vi "Rerun_GCFS.vi"() -> ()   [LabVIEW 2024]
uses:
  RerunCluster_GCFS.ctl
  <vilib>/userDefined/High Color/IMAQdx.ctl
  <vilib>/vision/Image Controls.llb/IMAQ Image.ctl
  <vilib>/Platform/TimedLoop/XDataNode/timing_clust.ctl
  <vilib>/Platform/TimedLoop/XDataNode/nitl_modes.ctl
  <vilib>/Platform/TimedLoop/XDataNode/wakeup.ctl
  <vilib>/addons/_JKI Toolkits/State Machine/_JKI_lib_State_Machine.llb/Select State(s)_err__jki_lib_state_machine.vi
  <extravilib>/ChannelInstances/Tag-t'RerunCluster_GCFS.ctl'/Read With Abort.vi
  <extravilib>/ChannelInstances/Stream-c(t'IMAQ Image.ctl',str,a[.,.](str),a[.,.](str),bool)/Read With Abort.vi
  <extravilib>/ChannelInstances/Stream-c(t'IMAQ Image.ctl',str,a[.,.](str),a[.,.](str),bool)/Write With Abort.vi
  <extravilib>/ChannelInstances/Tag-t'RerunCluster_GCFS.ctl'/Write With Abort.vi
  <extravilib>/ChannelInstances/Stream-c(t'IMAQ Image.ctl',str,a[.,.](str),a[.,.](str),bool)/EndpointRead.vi
  <extravilib>/ChannelInstances/Stream-c(t'IMAQ Image.ctl',str,a[.,.](str),a[.,.](str),bool)/Endpoint.vi
  <extravilib>/ChannelInstances/Stream-c(t'IMAQ Image.ctl',str,a[.,.](str),a[.,.](str),bool)/Instantiate.vi
  <extravilib>/ChannelInstances/Tag-t'RerunCluster_GCFS.ctl'/Instantiate.vi
  <extravilib>/ChannelInstances/Tag-t'RerunCluster_GCFS.ctl'/EndpointRead.vi
  <extravilib>/ChannelInstances/Stream-c(t'IMAQ Image.ctl',str,a[.,.](str),a[.,.](str),bool)/)Channel.vi
  <resource>/ChannelSupport/_ChannelSupport/WaitIfNeeded.vi
  <vilib>/addons/_JKI Toolkits/State Machine/_JKI_lib_State_Machine.llb/Periodic Trigger__ogtk__JKI-SM__jki_lib_state_machine.vi
  <vilib>/Utility/file.llb/Read Delimited Spreadsheet (DBL).vi
  <vilib>/Utility/file.llb/Read Delimited Spreadsheet (string).vi
  <extravilib>/ChannelInstances/Tag-t'RerunCluster_GCFS.ctl'/Endpoint.vi
  <vilib>/platform/TimedLoop/XDataNode/XDataNode.xnode
  <vilib>/regexp/Match Regular Expression.xnode
  <vilib>/Platform/TimedLoop/XDataNode/XDNodeRunTimeDep.lvlib
  <extravilib>/ChannelInstances/Stream-c(t'IMAQ Image.ctl',str,a[.,.](str),a[.,.](str),bool).lvlib
  <extravilib>/ChannelInstances/Tag-t'RerunCluster_GCFS.ctl'.lvlib
panel:
  out "Number of droplets":i32
  out "Droplet messurments":dbl[][](array[numeric])
  in  "Done":bool
  out "Timestamps and temp data":string[][](array[string])
  out "Sample Name":string
  out "Image":T1(plugin-control)
  in  "Active":bool
  in  "Load Rerun":bool
  out "Save loop":i32
  out "Frezz Image":T1(plugin-control)
  in  "Freezing value":sgl=250.0
  out "Temperature":dbl
  out "Data Loop":i32
  out "Statusstring":string
  in  "Exit":bool
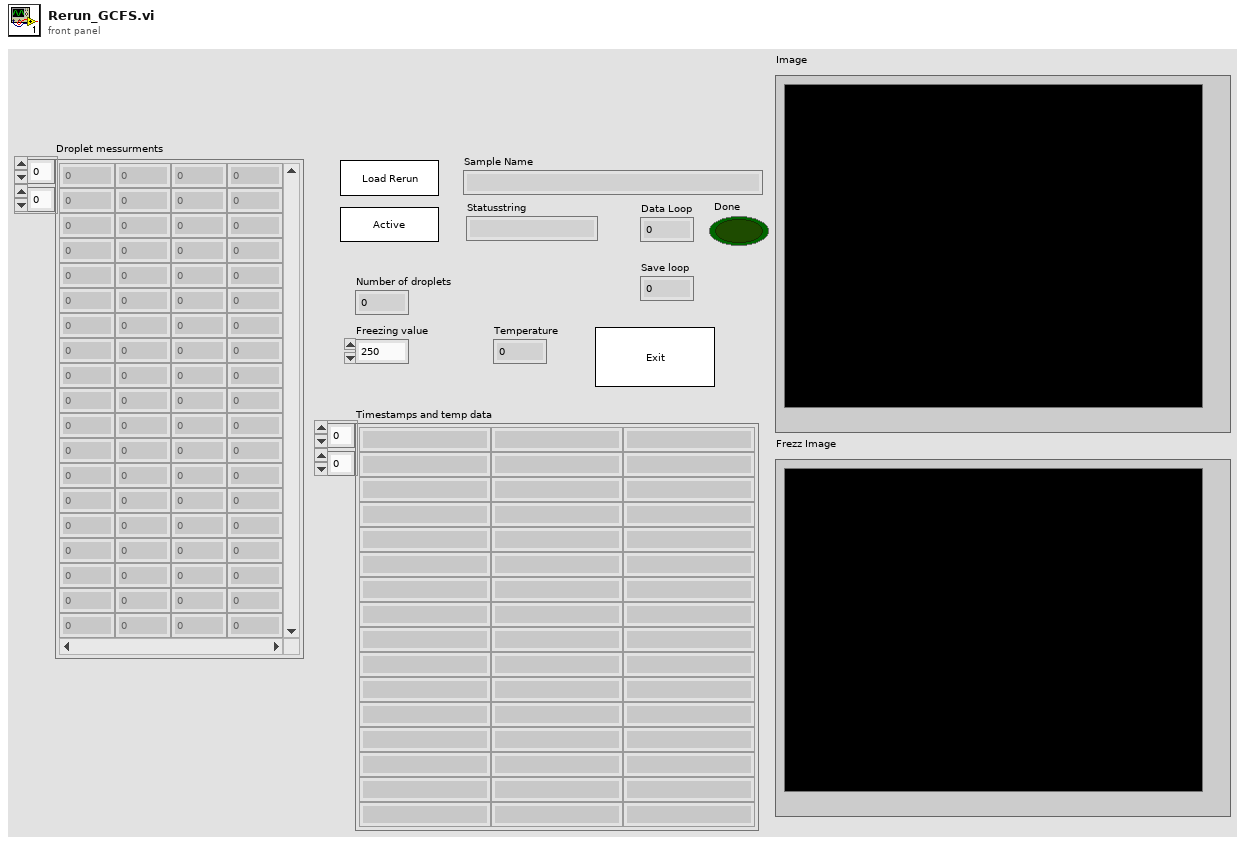
[diagram p1: front panel]
types:
  T1 = typedef "IMAQ Image.ctl" = refnum<image>
  T2 = typedef "RerunCluster_GCFS.ctl" = cluster{"Core":cluster{"Current VI Reference":refnum<vi>, "Close Panel on Exit?":bool}, "Your Boolean data":bool, "Your string data":string, "Camera Cluster":cluster{"Session":T3, "Image":T1, "Position Image":T1, "PixelVal Image":T1, "Position Image Rings":T1, "Lable Image":T1, "Merged Image":T1}, "Data In Cluster":cluster{"Images":cluster{"Position Image path":path, "Sample folder path":path, "Rerun Folder path":path, "Rerun pos.img. path":path}, "Sample Name":string, "Rerun Time":string, "Freezing value":sgl, "Number of images":i32}, "Active":bool, "Ready":bool, "Exit":bool, "Program_Start":string, "Data Out Cluster":cluster{"Particle Measurements":dbl[][], "Number of droplets":i32, "Time and temp":string[][], "Sample time (YYYY-MM-DD_hh;mm)":string}, "Load Rerun":bool, "Rerun":bool}
  T3 = typedef "IMAQdx.ctl" = refnum<k21>
  T4 = enum32{"Invalid", "Standard", "Closed", "Hidden", "Minimized", "Maximized"}
  T5 = enum32{"invalid app kind", "Development System", "Run Time System", "Student Edition", "Embedded LabVIEW", "Evaluation", "Custom"}
  T6 = cluster{"Left":i32, "Top":i32, "Right":i32, "Bottom":i32}
  T7 = cluster{"Current VI Reference":refnum<vi>, "Close Panel on Exit?":bool}
  T8 = typedef "Image Type" = u32
  T9 = typedef "Tag-t'RerunCluster_GCFS.ctl'.lvlib/))Channel.ctl" = refnum<queue>
  T10 = cluster{"Image To Save":T1, "Snap timestamp":string, "Pixel values":string[][], "Freezing points":string[][], "FreezingData":bool}
  T11 = typedef "XDNodeRunTimeDep.lvlib/timing_clust.ctl" = cluster{"Expected End [f-1]":u64, "Actual End [f-1]":u64, "Finished Late? [f-1]":bool, "Expected End [i-1]":u64, "Actual End [i-1]":u64, "Finished Late? [i-1]":bool, "Expected Start [i]":u64, "Actual Start [i]":u64, "Expected Start [f]":u64, "Actual Start [f]":u64, "Source Name":string, "Structure Name":string, "Period":i64, "Deadline":i64, "Offset":i64, "Start":i64, "Priority":i32, "Timeout":i32, "Mode":T12, "Wakeup Reason":T13, "Error":errorcluster, "Source Type":string, "Secondary Source Type":string, "Global End Time":u64, "Global Start Time":u64, "Frame Duration":u64, "Iteration Duration":u64, "Assigned CPU":i32, "I/O Scan Engine Mode":u32}
  T12 = typedef "XDNodeRunTimeDep.lvlib/nitl_modes.ctl" = enum32{"No Change", "Process missed periods, maintain original phase", "Discard missed periods, maintain original phase", "Process missed periods, ignore original phase", "Discard missed periods, ignore original phase"}
  T13 = typedef "XDNodeRunTimeDep.lvlib/wakeup.ctl" = enum32{"Normal", "Aborted", "Asynchronous wakeup", "Timing source error", "Timed loop error", "Timeout"}
  T14 = typedef "Stream-c(t'IMAQ Image.ctl',str,a[.,.](str),a[.,.](str),bool).lvlib/)Channel.ctl" = refnum<queue>
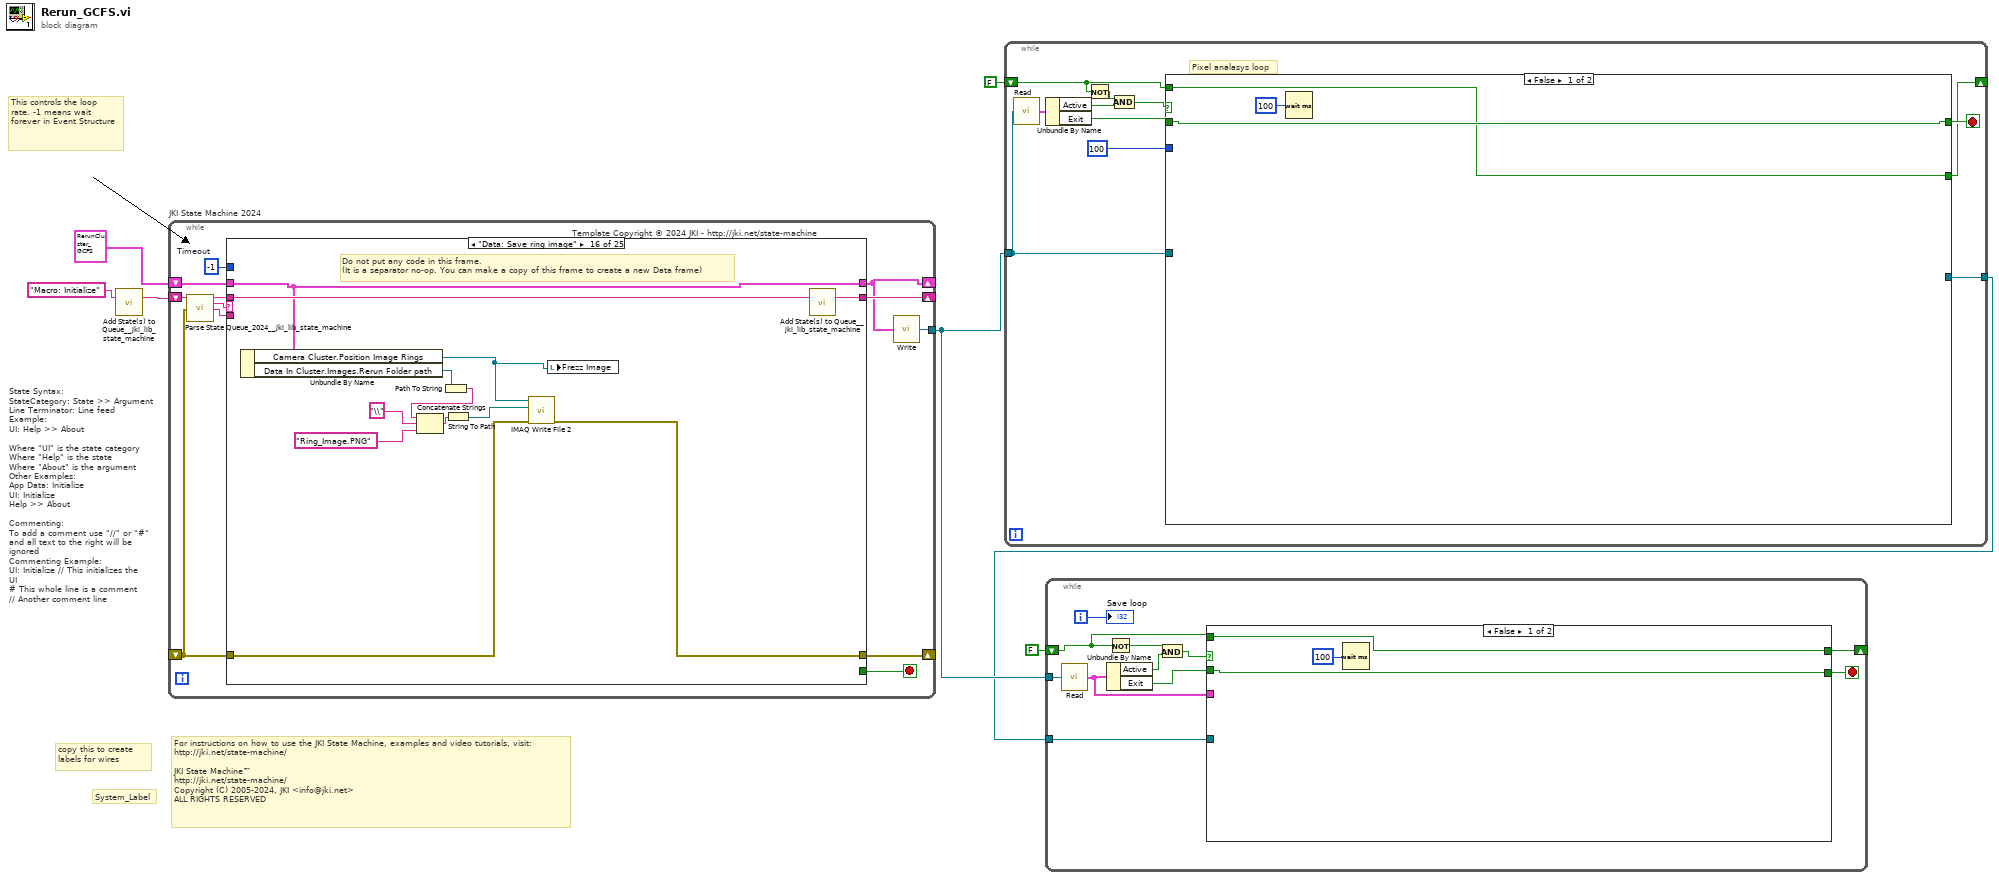
[diagram p0: block diagram]
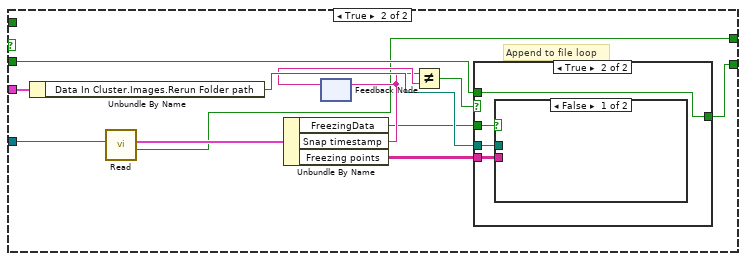
[diagram p2: hidden frame]
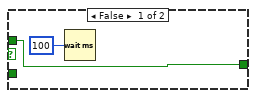
[diagram p3: hidden frame]
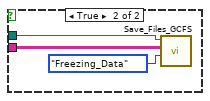
[diagram p4: hidden frame]
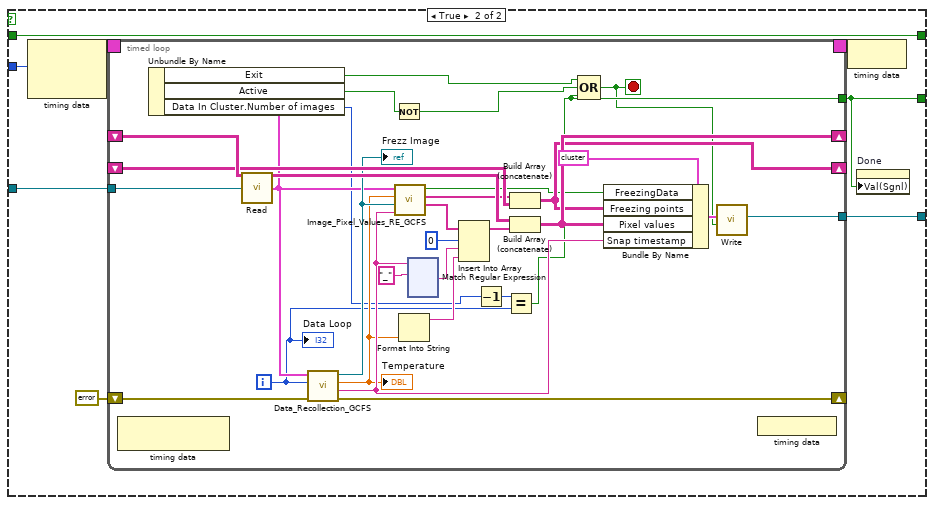
[diagram p5: hidden frame]
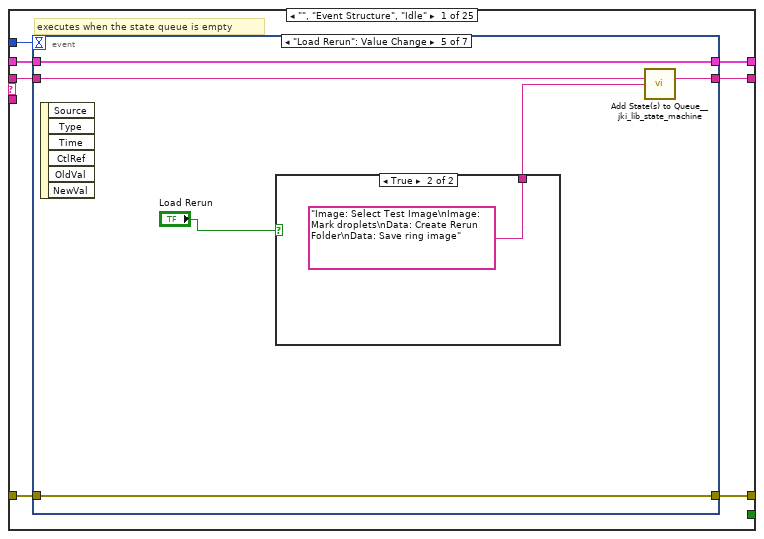
[diagram p6: hidden frame]
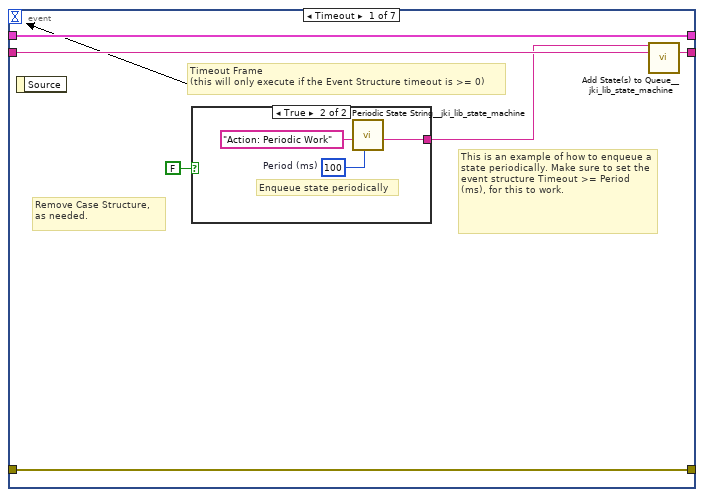
[diagram p7: hidden frame]
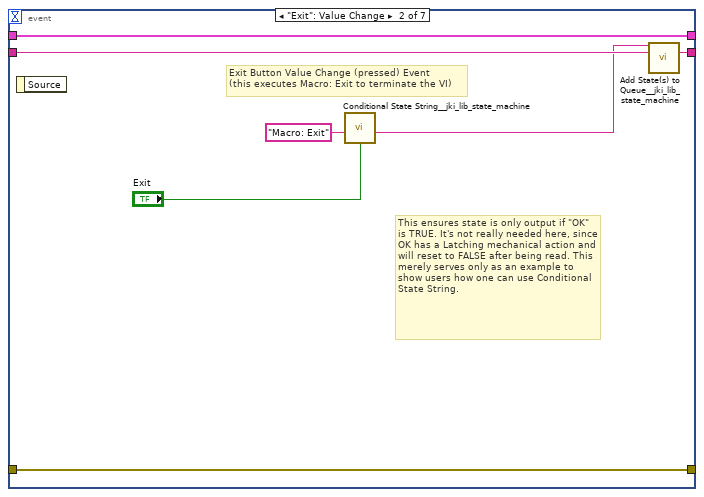
[diagram p9: hidden frame]
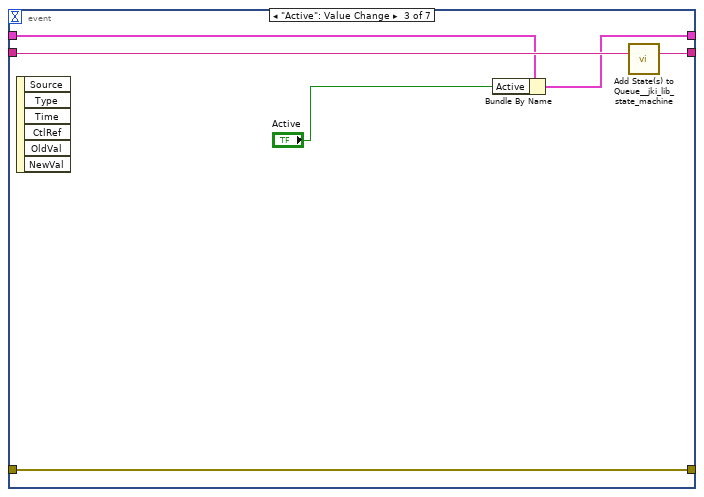
[diagram p10: hidden frame]
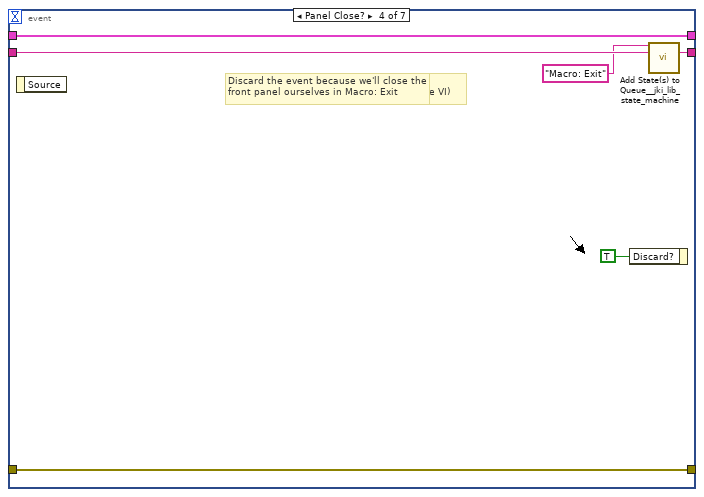
[diagram p11: hidden frame]
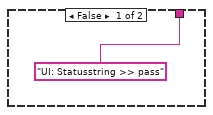
[diagram p12: hidden frame]
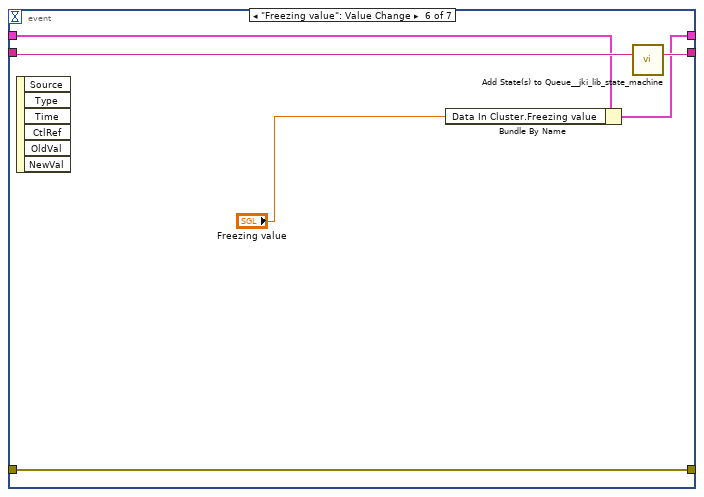
[diagram p13: hidden frame]
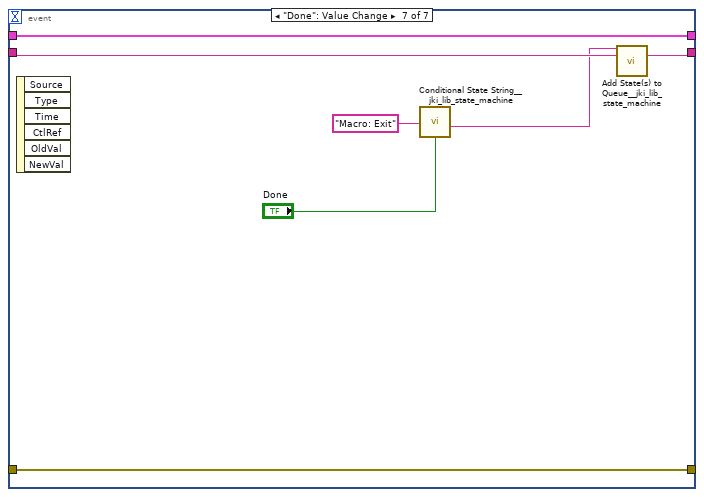
[diagram p14: hidden frame]
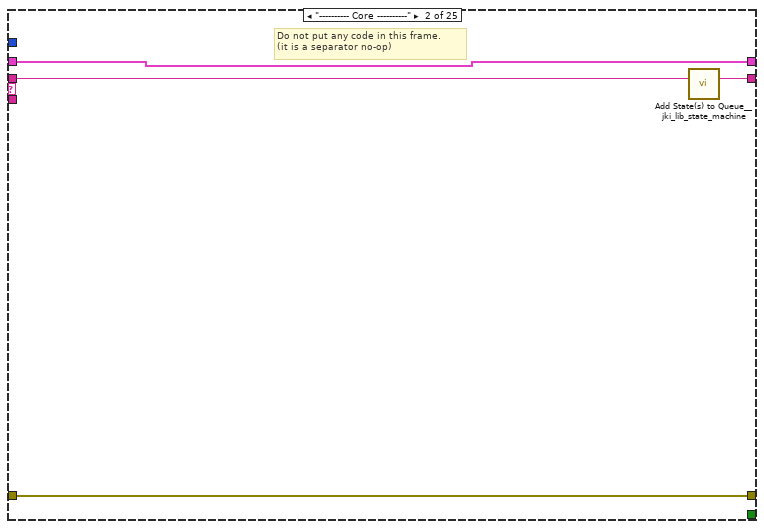
[diagram p15: hidden frame]
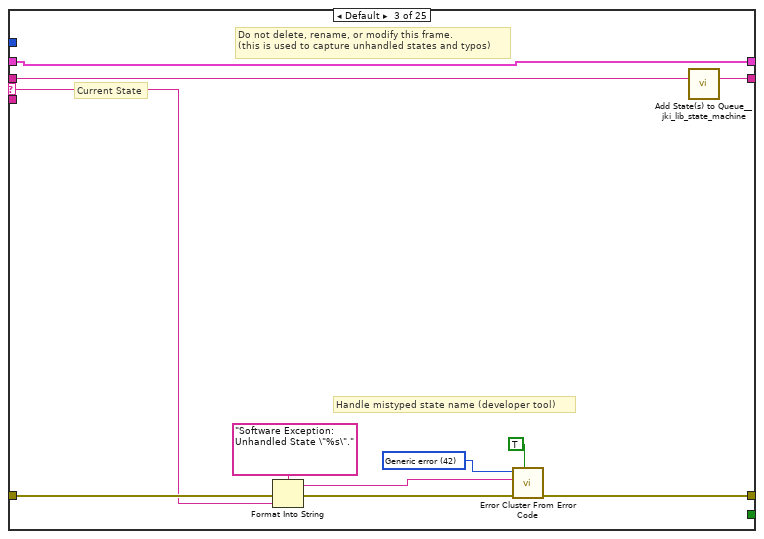
[diagram p16: hidden frame]
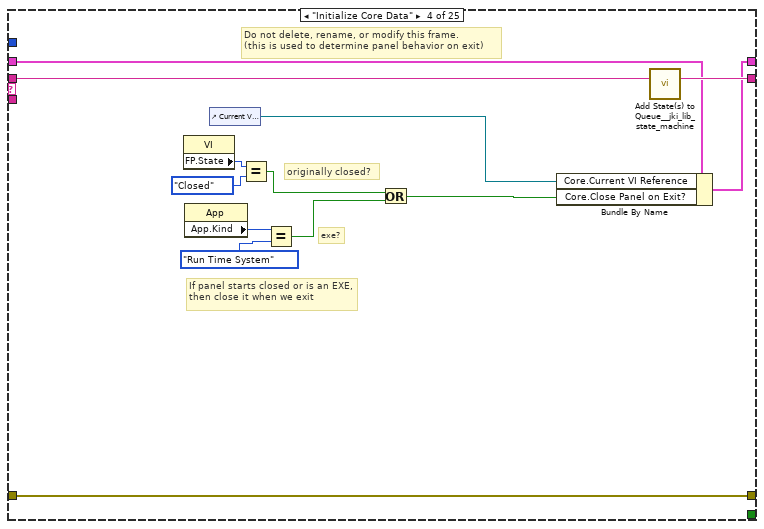
[diagram p17: hidden frame]
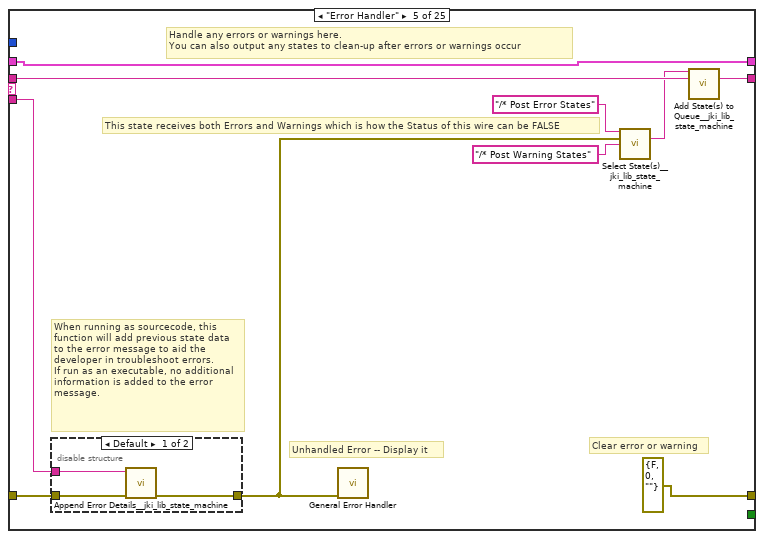
[diagram p18: hidden frame]
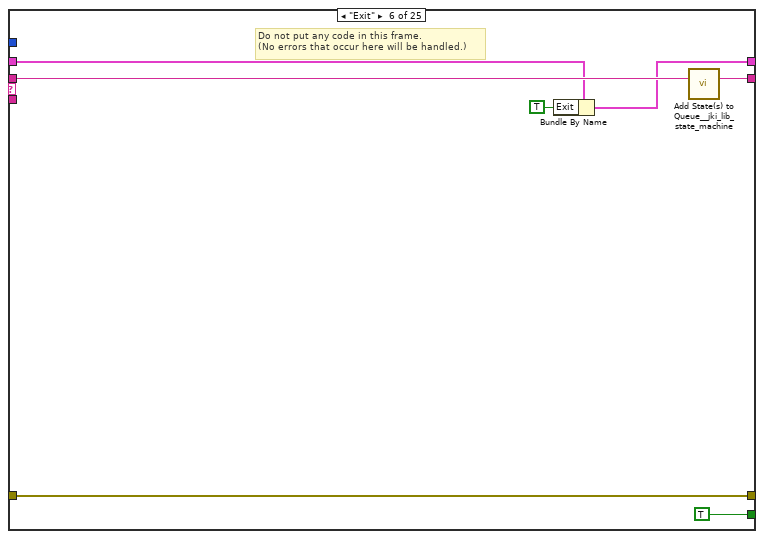
[diagram p20: hidden frame]
diagram:
  # "For instructions on how to use the JKI State Machine, examples and video tutorials, visit:\nhttp://jki.net/state-machine/\n\nJKI State Machine™\nhttp://jki.net/state-machine/\nCopyright (C) 2005-2024, JKI <info@jki.net>\nALL RIGHTS RESERVED"
  # "State Syntax:\nStateCategory: State >> Argument\nLine Terminator: Line feed\nExample:\nUI: Help >> About\n\nWhere \"UI\" is the state category\nWhere \"Help\" is the state\nWhere \"About\" is the argument\nOther Examples:\nApp Data: Initialize\nUI: Initialize\nHelp >> About\n\nCommenting:\nTo add a comment use \"//\" or \"#\" and all text to the right will be ignored\nCommenting Example:\nUI: Initialize // This initializes the UI\n# This whole line is a comment\n// Another comment line"
  # "copy this to create labels for wires"
  # "This controls the loop rate. -1 means wait forever in Event Structure"
  # "System_Label"
  n1 = call <vilib>:"Add State(s) to Queue__jki_lib_state_machine.vi"("State(s) in (\"\")"="Macro: Initialize") -> ("States Out"=w7:string)  [unwired: 14 in]
  n2 = while "JKI State Machine 2024" {
    shift-right: [w12] -> _
    shift-left: T2 {"Core"={"Current VI Reference"=refnum, "Close Panel on Exit?"=FALSE}, "Your Boolean data"=FALSE, "Your string data"="", "Camera Cluster"={"Session"="", "Image"=refnum, "Position Image"=refnum, "PixelVal Image"=refnum, "Position Image Rings"=refnum, "Lable Image"=refnum, "Merged Image"=refnum}, "Data In Cluster"={"Images"={"Position Image path"=path "", "Sample folder path"=path "", "Rerun Folder path"=path "", "Rerun pos.img. path"=path ""}, "Sample Name"="", "Rerun Time"="", "Freezing value"=250.0, "Number of images"=0}, "Active"=FALSE, "Ready"=FALSE, "Exit"=FALSE, "Program_Start"="", "Data Out Cluster"={"Particle Measurements"=[], "Number of droplets"=0, "Time and temp"=[], "Sample time (YYYY-MM-DD_hh;mm)"=""}, "Load Rerun"=FALSE, "Rerun"=FALSE} -> [w11]
    shift-right: [w15] -> _
    shift-left: _ -> [w9]
    shift-right: [w14] -> _
    shift-left: w7 -> [w16]
    tunnel: [w8] -> w5
    stop <- w13 stop-if-true
    w10 = -1  # Timeout
    # "Template Copyright © 2024 JKI - http://jki.net/state-machine"
    n3 = call <vilib>:"Parse State Queue_2024__jki_lib_state_machine.vi"("State Queue"=w16, "Error In (no error)"=w9) -> ("Remaining States"=w18:string, "Current State"=w19:string, "Arguments"=w17:string)  [unwired: 11 in]
    n4 = case shown="\"Data: Save ring image\"" w19 {
      selector: w19 -> [_ _ w80 _ _ _ _ _ _ _ _ _ _ _ _ _ _ _ _ _ _ _ _ _ _]
      tunnel: w18 -> [w26 w79 w84 w103 w113 w124 w128 w133 w144 w148 w175 w181 w200 w220 w235 w253 w257 w280 w291 w297 w308 w378 w382 w399 w409]
      tunnel: w17 -> [_ _ _ _ w108 _ _ _ _ _ _ _ _ _ _ _ _ _ _ w292 w302 w374 _ _ _]
      tunnel: w11 -> [w24 w76 w82 w96 w110 w120 w125 w130 w136 w145 w172 w176 w194 w214 w224 w251 w254 w278 w289 w295 w304 w375 w379 w385 w402]
      tunnel: [w23 w77 w86 w100 errorcluster {"status"=FALSE, "code"=0, "source"=""} ("error out") w122 w126 w131 w140 w146 w163 w177 w192 w211 w225 w246 w255 w272 w288 w293 w305 w376 w380 w390 w403] -> w15
      tunnel: w9 -> [w20 w77 w85 w100 w109 w122 w126 w131 w140 w146 w164 w178 w183 w212 w227 w247 w255 w274 w288 w294 w306 w376 w380 w386 w404]
      tunnel: [w25 w78 w83 w102 w112 w123 w127 w132 w143 w147 w174 w180 w199 w219 w234 w252 w256 w279 w290 w296 w307 w377 w381 w398 w408] -> w14
      tunnel: [_ _ _ _ _ TRUE _ _ _ _ _ _ _ _ _ _ _ _ _ _ _ _ _ _ _] -> w13
      tunnel: [w22 w76 w82 w101 w110 w119 w125 w130 w135 w145 w171 w176 w193 w213 w224 w251 w254 w278 w289 w295 w304 w375 w379 w397 w401] -> w12
      tunnel: w10 -> [w21 _ _ _ _ _ _ _ _ _ _ _ _ _ _ _ _ _ _ _ _ _ _ _ _]
      frame "", "Event Structure", "Idle" {
        # "executes when the state queue is empty"
        n5 = event shown="[4] \"Load Rerun\": Value Change" {
          selector: _ -> [_ _ _ _ _ _ _]
          dyn-events: _ -> [_ _ _ _ _ _ _]
          timeout: w21 -> [_ _ _ _ _ _ _]
          tunnel: w26 -> [w32 w42 w47 w54 w60 w67 w72]
          tunnel: [w31 w41 w48 w53 w59 w68 w73] -> w25
          tunnel: w24 -> [w29 w39 w46 w51 w55 w66 w75]
          tunnel: [w30 w40 w43 w52 w58 w63 w74] -> w23
          tunnel: w20 -> [w30 w40 w43 w52 w58 w63 w74]
          tunnel: [w29 w39 w45 w51 w55 w65 w75] -> w22
          event Timeout {
            # "Remove Case Structure, as needed."
            # "This is an example of how to enqueue a state periodically. Make sure to set the event structure Timeout >= Period (ms), for this to work."
            # "Timeout Frame\n(this will only execute if the Event Structure timeout is >= 0)"
            n6 = event-data() -> ()  [unwired: 1 in, 1 out]
            n7 = case shown="True" FALSE {
              tunnel: [_ w35] -> w28
              frame False {
              }
              frame True {
                w33 = u32 100  # Period (ms)
                # "Enqueue state periodically"
                n8 = call <vilib>:"Periodic State String__jki_lib_state_machine.vi"("Period (ms)"=w33, "State"="Action: Periodic Work") -> ("State Out"=w35:string)  [unwired: 9 in]
              }
            }
            n9 = call <vilib>:"Add State(s) to Queue__jki_lib_state_machine.vi"("State(s) in Front (\"\")"=w28, "State(s) in (\"\")"=w32) -> ("States Out"=w31:string)  [unwired: 13 in]
          }
          event "Exit": Value Change {
            # "This ensures state is only output if \"OK\" is TRUE. It's not really needed here, since OK has a Latching mechanical action and will reset to FALSE after being read. This merely serves only as an example to show users how one can use Conditional State String."
            # "Exit Button Value Change (pressed) Event\n(this executes Macro: Exit to terminate the VI)"
            n10 = event-data() -> ()  [unwired: 1 in, 1 out]
            n11 = call <vilib>:"Conditional State String__jki_lib_state_machine.vi"("Do State(s)?"="Exit", "State"="Macro: Exit") -> ("State Out"=w36:string)  [unwired: 7 in]
            n12 = call <vilib>:"Add State(s) to Queue__jki_lib_state_machine.vi"("State(s) in Front (\"\")"=w36, "State(s) in (\"\")"=w42) -> ("States Out"=w41:string)  [unwired: 13 in]
          }
          event "Active": Value Change {
            n13 = event-data() -> ()  [unwired: 1 in, 6 out]
            n14 = Bundle By Name(cluster=w46, "Active"="Active") -> (w45:T2)
            n15 = call <vilib>:"Add State(s) to Queue__jki_lib_state_machine.vi"("State(s) in (\"\")"=w47) -> ("States Out"=w48:string)  [unwired: 14 in]
          }
          event Panel Close? {
            # "Discard the event because we'll close the front panel ourselves in Macro: Exit"
            # "Close Panel button (pressed) Event\n(this executes Macro: Exit to terminate the VI)"
            n16 = event-data() -> ()  [unwired: 1 in, 1 out]
            n17 = event-data("Discard?"=TRUE) -> ()  [unwired: 1 in, 1 out]
            n18 = call <vilib>:"Add State(s) to Queue__jki_lib_state_machine.vi"("State(s) in Front (\"\")"="Macro: Exit", "State(s) in (\"\")"=w54) -> ("States Out"=w53:string)  [unwired: 13 in]
          }
          event "Load Rerun": Value Change {
            n19 = event-data() -> ()  [unwired: 1 in, 6 out]
            n20 = case shown="True" "Load Rerun" {
              tunnel: ["UI: Statusstring >> pass" "Image: Select Test Image\nImage: Mark droplets\nData: Create Rerun Folder\nData: Save ring image"] -> w57
              frame False {
              }
              frame True {
              }
            }
            n21 = call <vilib>:"Add State(s) to Queue__jki_lib_state_machine.vi"("State(s) in (\"\")"=w60, "State(s) at Back (\"\")"=w57) -> ("States Out"=w59:string)  [unwired: 13 in]
          }
          event "Freezing value": Value Change {
            n22 = event-data() -> ()  [unwired: 1 in, 6 out]
            n23 = Bundle By Name(cluster=w66, "Data In Cluster.Freezing value"="Freezing value") -> (w65:T2)
            n24 = call <vilib>:"Add State(s) to Queue__jki_lib_state_machine.vi"("State(s) in (\"\")"=w67) -> ("States Out"=w68:string)  [unwired: 14 in]
          }
          event "Done": Value Change {
            n25 = event-data() -> ()  [unwired: 1 in, 6 out]
            n26 = call <vilib>:"Conditional State String__jki_lib_state_machine.vi"("Do State(s)?"="Done", "State"="Macro: Exit") -> ("State Out"=w70:string)  [unwired: 7 in]
            n27 = call <vilib>:"Add State(s) to Queue__jki_lib_state_machine.vi"("State(s) in Front (\"\")"=w70, "State(s) in (\"\")"=w72) -> ("States Out"=w73:string)  [unwired: 13 in]
          }
        }
      }
      frame "---------- Core ----------" {
        # "Do not put any code in this frame.\n(it is a separator no-op)"
        n28 = call <vilib>:"Add State(s) to Queue__jki_lib_state_machine.vi"("State(s) in (\"\")"=w79) -> ("States Out"=w78:string)  [unwired: 14 in]
      }
      frame Default {
        w89 = 42 items=["No error", "Argument error", "Memory is full", "Out of zone", "End of file", "File already open", "Generic file I/O error", "File not found", "File permission error", "Disk is full", "Duplicate path", "Too many files open", "System feature not enabled", "Resource file not found", "Cannot add resource", "Resource not found", "Image not found", "Image memory error", "Pen does not exist", "Config type invalid", "Config token not found", "Config parse error", "Config memory error", "Bad external code format", "Bad external code offset", "External code not present", "Null window", "Destroy window error", "Null menu", "Print aborted", "Bad print record", "Print driver error", "Windows error during printing", "Memory error during printing", "Print dialog error", "Generic print error", "Invalid device refnum", "Device not found", "Device parameter error", "Device unit error", "Cannot open device", "Device call aborted", "Generic error", "Cancelled by user", "Object ID too low", "Object ID too high", "Object not in heap", "Unknown heap", "Unknown object (invalid DefProc)", "Unknown object (DefProc not in table)", "Message out of range", "Invalid (null) method", "Unknown message", "Manager call not supported", "Bad address", "Network operation in progress", "Network operation timed out", "Connection is busy", "Network attribute not supported", "Network error", "Address in use", "System out of memory", "Connection aborted", "Connection refused", "Not connected", "Already connected", "Connection closed", "Initialization error (interapplication manager)", "Bad occurrence", "Wait on unbound occurrence handler", "Occurrence queue overflow", "Datalog type conflict", "Unused", "Unrecognized type (interapplication manager)", "Memory corrupt", "Failed to make temporary DLL", "Old CIN version", "Drag socket not found", "Failed to load drop-object", "Failed to register OLE object", "Failed to release OLE object", "Format specifier type mismatch", "Unknown format specifier", "Too few format specifiers", "Too many format specifiers", "Scan failed", "Newer CIN version", "Error converting to variant", "Runtime menu error", "Password tampered", "Variant attribute not found", "Incompatible variant data type", "Event data is not available", "Event Store is not present", "Occurrence is not found", "Event Queue is not created", "Event info is not available", "Refnum passed is NULL", "Error retrieving Class GUID", "Error retrieving CoClass GUID", "Error retrieving TypeLib GUID.", "Bad built application magic bytes.", "Specific driver is different from the specific driver associated with the Logical Name.", "There is no session opened to the class driver.", "Max Error", "MAX - Error with config objects", "MAX - Error loading configuration", "MAX - Group not supported"]
        # "Current State"
        # "Do not delete, rename, or modify this frame.\n(this is used to capture unhandled states and typos)"
        # "Handle mistyped state name (developer tool)"
        n29 = Format Into String(format string="Software Exception: Unhandled State \"%s\"." ("message"), error in=w85, w80) -> (resulting string=w88:string, error out=w87:errorcluster)  [unwired: 1 in]
        n30 = call <vilib>:"Error Cluster From Error Code.vi"("show call chain? (False)"=TRUE, "error in (no error)"=w87, "error message (\"\")"=w88, "error code (0)"=w89) -> ("error out"=w86:errorcluster)  [unwired: 5 in]
        n31 = call <vilib>:"Add State(s) to Queue__jki_lib_state_machine.vi"("State(s) in (\"\")"=w84) -> ("States Out"=w83:string)  [unwired: 14 in]
      }
      frame "Initialize Core Data" {
        # "Do not delete, rename, or modify this frame.\n(this is used to determine panel behavior on exit)"
        # "originally closed?"
        # "exe?"
        # "If panel starts closed or is an EXE, then close it when we exit"
        n32 = property class="VI"() -> ("FP.State"=w93:T4)  [unwired: 2 in, 2 out]
        n33 = property class="App"() -> ("App.Kind"=w99:T5)  [unwired: 2 in, 2 out]
        n34 = control-ref of="Current VI Reference"() -> (w94:refnum<vi>)
        n35 = Equal?(x=w93, y=T4."Closed" ("Front Panel Window:State")) -> (x = y?=w91:bool)
        n36 = Equal?(x=w99, y=T5."Run Time System" ("Application:Kind")) -> (x = y?=w97:bool)
        n37 = Or(x=w91, y=w97) -> (x .or. y?=w95:bool)
        n38 = Bundle By Name(cluster=w96, "Core.Current VI Reference"=w94, "Core.Close Panel on Exit?"=w95) -> (w101:T2)
        n39 = call <vilib>:"Add State(s) to Queue__jki_lib_state_machine.vi"("State(s) in (\"\")"=w103) -> ("States Out"=w102:string)  [unwired: 14 in]
      }
      frame "Error Handler" {
        # "When running as sourcecode, this function will add previous state data to the error message to aid the developer in troubleshoot errors.\nIf run as an executable, no additional information is added to the error message."
        # "This state receives both Errors and Warnings which is how the Status of this wire can be FALSE"
        # "Unhandled Error -- Display it"
        # "Handle any errors or warnings here.\nYou can also output any states to clean-up after errors or warnings occur"
        # "Clear error or warning"
        n40 = disable-structure shown="Default" {
          disable-tunnel: w109 -> [w116 w117]
          disable-tunnel: w108 -> [w115 _]
          disable-tunnel: [w114 w117] -> w107
          frame condition #0 (active) {
            n41 = call <vilib>:"Append Error Details__jki_lib_state_machine.vi"("error in (no error)"=w116, "Previous State and Argument(s)"=w115) -> ("error out"=w114:errorcluster)  [unwired: 9 in]
          }
          frame condition #1 {
          }
        }
        n42 = call <vilib>:"General Error Handler.vi"("error in (no error)"=w107) -> ()  [unwired: 10 in, 5 out]
        n43 = call-poly <vilib>:"Select State(s)__jki_lib_state_machine.vi"("State(s) if True (\"\")"="/* Post Error States", "Select"=w107, "State(s) if False (\"\")"="/* Post Warning States") -> ("States Out"=w105:string)  [unwired: 12 in]
        n44 = call <vilib>:"Add State(s) to Queue__jki_lib_state_machine.vi"("State(s) in Front (\"\")"=w105, "State(s) in (\"\")"=w113) -> ("States Out"=w112:string)  [unwired: 13 in]
      }
      frame "Exit" {
        # "Do not put any code in this frame.\n(No errors that occur here will be handled.)"
        n45 = Bundle By Name(cluster=w120, "Exit"=TRUE) -> (w119:T2)
        n46 = call <vilib>:"Add State(s) to Queue__jki_lib_state_machine.vi"("State(s) in (\"\")"=w124) -> ("States Out"=w123:string)  [unwired: 14 in]
      }
      frame "---------- Macro ----------" {
        # "Do not put any code in this frame.\n(It is a separator no-op. You can make a copy of this frame to create a new Macro frame)"
        n47 = call <vilib>:"Add State(s) to Queue__jki_lib_state_machine.vi"("State(s) in (\"\")"=w128) -> ("States Out"=w127:string)  [unwired: 14 in]
      }
      frame "Macro: Initialize" {
        w129 = "Data: Initialize\nUI: Initialize\nData: Pull droplet data\nData: Pull timestamps and temp data\nInitialize Core Data\nUI: Statusstring >> Initialysing\nUI: Front Panel State >> Open\nUI: Statusstring >> Initialysation done\n"  # Data: Initialize UI: Initialize Data: Pull droplet data Data: Pull timestamps and temp data Initialize Core Data UI: Statusstring >> Initialysing UI: Front Panel State >> Open UI: Statusstring >> Initialysation done
        # "Initialization Macro\n(This is called once, when the VI starts)"
        n48 = call <vilib>:"Add State(s) to Queue__jki_lib_state_machine.vi"("State(s) in Front (\"\")"=w129, "State(s) in (\"\")"=w133) -> ("States Out"=w132:string)  [unwired: 13 in]
      }
      frame "Macro: Exit" {
        w134 = FALSE ("Active")
        # "Exit Macro\n(This is called once, when the VI exits)"
        n49 = Unbundle By Name(w136) -> ("Core.Close Panel on Exit?"=w138:bool)
        n50 = property on="Active" class="Bool (strict)"("Value"=w134) -> ()  [unwired: 2 in, 2 out]
        n51 = call <vilib>:"Conditional State String__jki_lib_state_machine.vi"("Do State(s)?"=w138, "State"="UI: Front Panel State >> Close") -> ("State Out"=w137:string)  [unwired: 7 in]
        n52 = Bundle By Name(cluster=w136, "Active"=w134) -> (w135:T2)
        n53 = call <vilib>:"Add State(s) to Queue__jki_lib_state_machine.vi"("State(s) in (\"\")"=w137, "State(s) at Back (\"\")"="UI: Uninitialize\nData: Cleanup\nExit") -> ("States Out"=w141:string)  [unwired: 13 in]
        n54 = call <vilib>:"Add State(s) to Queue__jki_lib_state_machine.vi"("State(s) in Front (\"\")"=w141, "State(s) in (\"\")"=w144) -> ("States Out"=w143:string)  [unwired: 13 in]
      }
      frame "---------- Data ----------" {
        # "Do not put any code in this frame.\n(It is a separator no-op. You can make a copy of this frame to create a new Data frame)"
        n55 = call <vilib>:"Add State(s) to Queue__jki_lib_state_machine.vi"("State(s) in (\"\")"=w148) -> ("States Out"=w147:string)  [unwired: 14 in]
      }
      frame "Data: Initialize" {
        w166 = "\\" ("string")
        w173 = T7 {"Current VI Reference"=refnum, "Close Panel on Exit?"=FALSE}  # Core
        # "Select Position Image in sample folder"
        # "do not delete - used by framework"
        # "Initialize the shift-register data, here.\n(data names are defined by what you wire into the bundle function)"
        n56 = call <vilib>:"Application Directory.vi"() -> ("Application Directory"=w168:path)
        n57 = Path To String(path=w168) -> (string=w167:string)
        n58 = Concatenate Strings(w167, w166, "Flat Surface Images" ("string"), w166) -> (w160:string)
        n59 = String To Path(string=w160) -> (path=w165:path)
        n60 = call "File Dialog2"("start path"=w165, "prompt"="Select Position image in sample folder", "error in"=w164, "pattern (all files)"="*.png*") -> ("selected path"=w151:path, "error out"=w163:errorcluster)  [unwired: 8 in, 2 out]
        n61 = Path To String(path=w151) -> (string=w161:string)
        n62 = Search and Replace String(input string=w161, search string=w160) -> (result string=w158:string)  [unwired: 6 in, 3 out]
        n63 = Match Pattern(string=w158, regular expression="\\" ("search string/char (-)")) -> (before substring=w149:string, match substring=w155:string, after substring=w156:string)  [unwired: 1 in, 1 out]
        "Sample Name" <- w149
        n64 = Match Pattern(string=w156, regular expression="\\" ("search string/char (-)")) -> (before substring=w150:string)  [unwired: 1 in, 3 out]
        n65 = Concatenate Strings(w149, w155, w150) -> (w154:string)
        n66 = Concatenate Strings(w160, w154) -> (w153:string)
        n67 = String To Path(string=w153) -> (path=w152:path)
        n68 = Bundle By Name(cluster=w172, "Core"=w173, "Data In Cluster.Sample Name"=w149, "Data In Cluster.Images.Sample folder path"=w152, "Data In Cluster.Images.Rerun pos.img. path"=w151, "Data Out Cluster.Sample time (YYYY-MM-DD_hh;mm)"=w150) -> (w171:T2)
        n69 = call <vilib>:"Add State(s) to Queue__jki_lib_state_machine.vi"("State(s) in (\"\")"=w175) -> ("States Out"=w174:string)  [unwired: 14 in]
      }
      frame "Data: Cleanup" {
        # "Cleanup any data and references, here.\n(this is called automatically, by the Macro: Exit)"
        n70 = Unbundle By Name(w176) -> ("Core.Current VI Reference"=w179:refnum<vi>)
        n71 = Close Reference(reference=w179, error in (no error)=w178) -> (error out=w177:errorcluster)
        n72 = call <vilib>:"Add State(s) to Queue__jki_lib_state_machine.vi"("State(s) in (\"\")"=w181) -> ("States Out"=w180:string)  [unwired: 14 in]
      }
      frame "Data: Pull droplet data" {
        n73 = Unbundle By Name(w194) -> ("Data In Cluster.Images.Sample folder path"=w198:path)
        n74 = Path To String(path=w198) -> (string=w191:string)
        n75 = Concatenate Strings(w191, "\\" ("search string/char (-)"), "Droplet_data.csv" ("string")) -> (w196:string)
        n76 = String To Path(string=w196) -> (path=w195:path)
        n77 = call-poly <vilib>:"Read Delimited Spreadsheet.vi"("file path (dialog if empty)"=w195, "error in (no error)"=w183, "delimiter (\\t)"=";" ("delimiter (\\t)")) -> ("all rows"=w185:dbl[][], "error out"=w192:errorcluster)  [unwired: 7 in, 4 out]
        n78 = Delete From Array(array=w185, index (row)=0) -> (array with subset deleted=w184:dbl[][])  [unwired: 2 in, 1 out]
        "Droplet messurments" <- w184
        n79 = Index Array(array=w184, index (col)=0 ("disabled index (col)")) -> (element=w188:dbl[])  [unwired: 1 in]
        n80 = Array Size(array=w188) -> (size(s)=w187:i32)
        "Number of droplets" <- w187
        n81 = Bundle By Name(cluster=w194, "Data Out Cluster.Particle Measurements"=w184, "Data Out Cluster.Number of droplets"=w187) -> (w193:T2)
        n82 = call <vilib>:"Add State(s) to Queue__jki_lib_state_machine.vi"("State(s) in (\"\")"=w200) -> ("States Out"=w199:string)  [unwired: 14 in]
      }
      frame "Data: Pull timestamps and temp data" {
        n83 = Unbundle By Name(w214) -> ("Data In Cluster.Images.Sample folder path"=w218:path)
        n84 = Path To String(path=w218) -> (string=w209:string)
        n85 = Concatenate Strings(w209, "\\" ("search string/char (-)"), "Sample_data.csv" ("string")) -> (w216:string)
        n86 = String To Path(string=w216) -> (path=w215:path)
        n87 = call-poly <vilib>:"Read Delimited Spreadsheet.vi"("file path (dialog if empty)"=w215, "format (%s)"="%s", "number of rows (all:-1)"=3, "error in (no error)"=w212, "transpose? (F)"=TRUE, "delimiter (\\t)"=";" ("delimiter (\\t)")) -> ("all rows"=w204:string[][], "error out"=w211:errorcluster)  [unwired: 4 in, 4 out]
        "Timestamps and temp data" <- w204
        n88 = Index Array(array=w204, index (col)=0 ("disabled index (col)")) -> (element=w202:string[])  [unwired: 1 in]
        n89 = Array Size(array=w202) -> (size(s)=w201:i32)
        n90 = Bundle By Name(cluster=w214, "Data Out Cluster.Time and temp"=w204, "Data In Cluster.Number of images"=w201) -> (w213:T2)
        n91 = call <vilib>:"Add State(s) to Queue__jki_lib_state_machine.vi"("State(s) in (\"\")"=w220) -> ("States Out"=w219:string)  [unwired: 14 in]
      }
      frame "Data: Create Rerun Folder" {
        n92 = Unbundle By Name(w224) -> ("Data In Cluster.Images.Sample folder path"=w233:path, "Data In Cluster.Rerun Time"=w232:string)
        n93 = Path To String(path=w233) -> (string=w222:string)
        n94 = Concatenate Strings(w222, "\\" ("search string/char (-)"), w232) -> (w231:string)
        n95 = String To Path(string=w231) -> (path=w230:path)
        n96 = call <vilib>:"Check if File or Folder Exists.vi"("error in (no error)"=w227, "path"=w230) -> ("error out"=w226:errorcluster, "file or folder exists?"=w229:bool, "dup path"=w228:path)  [unwired: 7 in]
        n97 = case shown="False" w229 {
          tunnel: w228 -> [w239 w241]
          tunnel: [w238 w241] -> w223
          tunnel: [w237 w240] -> w225
          tunnel: w226 -> [w236 w240]
          frame False {
            n98 = Create Folder(path (use dialog)=w239, error in=w236) -> (created path=w238:path, error out=w237:errorcluster)  [unwired: 1 in, 1 out]
          }
          frame True {
          }
        }
        n99 = Bundle By Name(cluster=w224, "Data In Cluster.Images.Rerun Folder path"=w223) -> ()  [unwired: 1 out]
        n100 = call <vilib>:"Add State(s) to Queue__jki_lib_state_machine.vi"("State(s) in (\"\")"=w235) -> ("States Out"=w234:string)  [unwired: 14 in]
      }
      frame "Data: Save ring image" {
        # "Do not put any code in this frame.\n(It is a separator no-op. You can make a copy of this frame to create a new Data frame)"
        n101 = Unbundle By Name(w251) -> ("Camera Cluster.Position Image Rings"=w243:T1, "Data In Cluster.Images.Rerun Folder path"=w242:path)
        n102 = Path To String(path=w242) -> (string=w250:string)
        n103 = Concatenate Strings(w250, "\\" ("string"), "Ring_Image.PNG" ("string")) -> (w249:string)
        n104 = String To Path(string=w249) -> (path=w248:path)
        n105 = call-poly "IMAQ Write File 2"("error in (no error)"=w247, "File Path"=w248, "Image"=w243) -> ("error out"=w246:errorcluster)  [unwired: 7 in, 1 out]
        n106 = local write "Frezz Image"(w243) -> ()
        n107 = call <vilib>:"Add State(s) to Queue__jki_lib_state_machine.vi"("State(s) in (\"\")"=w253) -> ("States Out"=w252:string)  [unwired: 14 in]
      }
      frame "---------- UI ----------" {
        # "Do not put any code in this frame.\n(It is a separator no-op. You can make a copy of this frame to create a new UI frame)"
        n108 = call <vilib>:"Add State(s) to Queue__jki_lib_state_machine.vi"("State(s) in (\"\")"=w257) -> ("States Out"=w256:string)  [unwired: 14 in]
      }
      frame "UI: Initialize" {
        w260 = FALSE ("Cool")
        w268 = "\\" ("string")
        w276 = T8 6 items=["Grayscale (U8)", "Grayscale (I16)", "Grayscale (SGL)", "Complex (CSG)", "RGB (U32)", "HSL (U32)", "RGB (U64)", "Grayscale (U16)"] ("Image Type")
        w264 = T1 refnum ("Image")
        # "Initialize the User Interface, here.\n(this is called automatically, by the Macro: Initialize)"
        n109 = call <vilib>:"Application Directory.vi"() -> ("Application Directory"=w271:path)
        n110 = Path To String(path=w271) -> (string=w270:string)
        n111 = Concatenate Strings(w270, w268, "resources" ("string"), w268, "Logo_Full.png" ("string")) -> (w266:string)
        n112 = String To Path(string=w266) -> (path=w265:path)
        n113 = local write "Image"(w264) -> ()
        n114 = local write "Frezz Image"(w264) -> ()
        n115 = call "IMAQ Create"("Image Name"="Logo", "Image Type"=w276, "error in (no error)"=w274) -> ("New Image"=w275:T1, "error out"=w273:errorcluster)  [unwired: 2 in]
        n116 = local write "Data Loop"(0 ("Data Loop")) -> ()
        n117 = call "IMAQ ReadFile 2"("File Path"=w265, "error in (no error)"=w273, "Image"=w275) -> ("error out"=w272:errorcluster)  [unwired: 4 in, 4 out]
        n118 = local write "Done"(w260) -> ()
        n119 = property on="Active" class="Bool (strict)"("Value"=w260) -> ()  [unwired: 2 in, 2 out]
        n120 = local write "Number of droplets"(0 ("Number of droplets")) -> ()
        n121 = local write "Droplet messurments"(dbl[][] [] ("Droplet messurments")) -> ()
        n122 = property on="Temperature" class="DigNum (strict)"("Value"=0.0 ("Temperature")) -> ()  [unwired: 2 in, 2 out]
        n123 = local write "Timestamps and temp data"(string[][] [] ("Timestamps and temp data")) -> ()
        n124 = call <vilib>:"Add State(s) to Queue__jki_lib_state_machine.vi"("State(s) in (\"\")"=w280) -> ("States Out"=w279:string)  [unwired: 14 in]
      }
      frame "UI: Uninitialize" {
        w284 = T1 refnum ("Image")
        # "Cleanup the User Interface, here.\n(this is called automatically, by the Macro: Exit)"
        n125 = local write "Image"(w284) -> ()
        n126 = local write "Frezz Image"(w284) -> ()
        n127 = local write "Data Loop"(0 ("Data Loop")) -> ()
        n128 = property on="Active" class="Bool (strict)"("Value"=FALSE ("Cool")) -> ()  [unwired: 2 in, 2 out]
        n129 = property on="Temperature" class="DigNum (strict)"("Value"=0.0 ("Temperature")) -> ()  [unwired: 2 in, 2 out]
        n130 = local write "Timestamps and temp data"(string[][] [] ("Timestamps and temp data")) -> ()
        n131 = local write "Number of droplets"(0 ("Number of droplets")) -> ()
        n132 = local write "Droplet messurments"(dbl[][] [] ("Droplet messurments")) -> ()
        n133 = call <vilib>:"Add State(s) to Queue__jki_lib_state_machine.vi"("State(s) in (\"\")"=w291) -> ("States Out"=w290:string)  [unwired: 14 in]
      }
      frame "UI: Cursor Set" {
        # "Argument"
        # "Set and Unset Cursor Busy.\n(Usage: \"UI: Cursor Set >> Busy|Idle\")"
        n134 = case shown="\"Idle\", Default" w292 {
          tunnel: w294 -> [w299 w301]
          tunnel: [w298 w300] -> w293
          frame "Idle", Default {
            n135 = call <vilib>:"Unset Busy.vi"("error in (no error)"=w299) -> ("error out"=w298:errorcluster)  [unwired: 10 in]
          }
          frame "Busy" {
            n136 = call <vilib>:"Set Busy.vi"("error in (no error)"=w301) -> ("error out"=w300:errorcluster)  [unwired: 9 in, 1 out]
          }
        }
        n137 = call <vilib>:"Add State(s) to Queue__jki_lib_state_machine.vi"("State(s) in (\"\")"=w297) -> ("States Out"=w296:string)  [unwired: 14 in]
      }
      frame "UI: Front Panel State" {
        # "Argument"
        # "Set Front Panel Open or Closed\n(Usage: \"UI: Front Panel State >> Open|Close\")"
        n138 = Unbundle By Name(w304) -> ("Core.Current VI Reference"=w303:refnum<vi>)
        n139 = case shown="\"Open\", \"Standard\", Default" w302 {
          tunnel: w306 -> [w314 w329 w340 w353 w366]
          tunnel: [w316 w330 w342 w355 w368] -> w305
          tunnel: w303 -> [w315 w327 w341 w354 w367]
          frame "Open", "Standard", Default {
            w309 = T4."Standard" ("State")
            n140 = property class="VI"(reference=w315, error in=w314) -> (reference out=w312:refnum<vi>, error out=w313:errorcluster, "FP.State"=w311:T4)
            n141 = Not Equal?(x=w311, y=w309) -> (x != y?=w310:bool)
            n142 = case shown="False" w310 {
              tunnel: [w320 w322] -> w316
              tunnel: w313 -> [w319 w322]
              tunnel: w312 -> [w318 _]
              tunnel: w309 -> [w317 _]
              frame True {
                n143 = invoke class="VI" method="FP.Open"(reference=w318, error in=w319, "Activate"=TRUE, "State"=w317) -> (error out=w320:errorcluster)  [unwired: 1 in, 4 out]
              }
              frame False {
              }
            }
          }
          frame "Close", "Closed" {
            n144 = property class="VI"(reference=w327, error in=w329) -> (reference out=w326:refnum<vi>, error out=w328:errorcluster, "FP.State"=w324:T4)
            n145 = Not Equal?(x=w324, y=T4."Closed" ("Front Panel Window:State")) -> (x != y?=w323:bool)
            n146 = case shown="True" w323 {
              tunnel: [w331 w334] -> w330
              tunnel: w328 -> [w331 w333]
              tunnel: w326 -> [_ w332]
              frame False {
              }
              frame True {
                n147 = invoke class="VI" method="FP.Close"(reference=w332, error in=w333) -> (error out=w334:errorcluster)  [unwired: 1 in, 2 out]
              }
            }
          }
          frame "Hidden", "Hide" {
            w335 = T4."Hidden" ("State")
            n148 = property class="VI"(reference=w341, error in=w340) -> (reference out=w338:refnum<vi>, error out=w339:errorcluster, "FP.State"=w337:T4)
            n149 = Not Equal?(x=w337, y=w335) -> (x != y?=w336:bool)
            n150 = case shown="True" w336 {
              tunnel: [w346 w347] -> w342
              tunnel: w339 -> [w345 w347]
              tunnel: w338 -> [w344 _]
              tunnel: w335 -> [w343 _]
              frame True {
                n151 = invoke class="VI" method="FP.Open"(reference=w344, error in=w345, "State"=w343) -> (error out=w346:errorcluster)  [unwired: 2 in, 4 out]
              }
              frame False {
              }
            }
          }
          frame "Minimize", "Minimized" {
            w348 = T4."Minimized" ("State")
            n152 = property class="VI"(reference=w354, error in=w353) -> (reference out=w351:refnum<vi>, error out=w352:errorcluster, "FP.State"=w350:T4)
            n153 = Not Equal?(x=w350, y=w348) -> (x != y?=w349:bool)
            n154 = case shown="True" w349 {
              tunnel: [w359 w360] -> w355
              tunnel: w352 -> [w358 w360]
              tunnel: w351 -> [w357 _]
              tunnel: w348 -> [w356 _]
              frame True {
                n155 = invoke class="VI" method="FP.Open"(reference=w357, error in=w358, "State"=w356) -> (error out=w359:errorcluster)  [unwired: 2 in, 4 out]
              }
              frame False {
              }
            }
          }
          frame "Maximize", "Maximized" {
            w361 = T4."Maximized" ("State")
            n156 = property class="VI"(reference=w367, error in=w366) -> (reference out=w364:refnum<vi>, error out=w365:errorcluster, "FP.State"=w363:T4)
            n157 = Not Equal?(x=w363, y=w361) -> (x != y?=w362:bool)
            n158 = case shown="True" w362 {
              tunnel: [w372 w373] -> w368
              tunnel: w365 -> [w371 w373]
              tunnel: w364 -> [w370 _]
              tunnel: w361 -> [w369 _]
              frame True {
                n159 = invoke class="VI" method="FP.Open"(reference=w370, error in=w371, "State"=w369) -> (error out=w372:errorcluster)  [unwired: 2 in, 4 out]
              }
              frame False {
              }
            }
          }
        }
        n160 = call <vilib>:"Add State(s) to Queue__jki_lib_state_machine.vi"("State(s) in (\"\")"=w308) -> ("States Out"=w307:string)  [unwired: 14 in]
      }
      frame "UI: Statusstring" {
        # "Do not put any code in this frame.\n(It is a separator no-op. You can make a copy of this frame to create a new UI frame)"
        n161 = call <vilib>:"Add State(s) to Queue__jki_lib_state_machine.vi"("State(s) in (\"\")"=w378) -> ("States Out"=w377:string)  [unwired: 14 in]
        "Statusstring" <- w374
      }
      frame "---------- Image ----------" {
        # "Template Separator\n(You can make a copy of, or modify, this frame)"
        n162 = call <vilib>:"Add State(s) to Queue__jki_lib_state_machine.vi"("State(s) in (\"\")"=w382) -> ("States Out"=w381:string)  [unwired: 14 in]
      }
      frame "Image: Select Test Image" {
        w393 = T8 1 items=["Grayscale (U8)", "Grayscale (I16)", "Grayscale (SGL)", "Complex (CSG)", "RGB (U32)", "HSL (U32)", "RGB (U64)", "Grayscale (U16)"] ("Image Type")
        # "Template Separator\n(You can make a copy of, or modify, this frame)"
        n163 = Unbundle By Name(w385) -> ("Data In Cluster.Images.Rerun pos.img. path"=w384:path)
        n164 = call "IMAQ Create"("Image Name"="Position", "Image Type"=w393, "error in (no error)"=w386) -> ("New Image"=w392:T1, "error out"=w391:errorcluster)  [unwired: 2 in]
        n165 = Format Date/Time String(time format string (%c)="%Y-%m-%d_%H;%M;%S", UTC format=FALSE) -> (date/time string=w389:string)  [unwired: 1 in]
        n166 = call "IMAQ ReadFile 2"("File Path"=w384, "error in (no error)"=w391, "Image"=w392) -> ("error out"=w390:errorcluster, "Image Out"=w383:T1)  [unwired: 4 in, 3 out]
        "Image" <- w383
        n167 = Concatenate Strings("RERUN_" ("string"), w389) -> (w387:string)
        n168 = Bundle By Name(cluster=w385, "Camera Cluster.Image"=w383, "Data In Cluster.Rerun Time"=w387) -> (w397:T2)
        n169 = call <vilib>:"Add State(s) to Queue__jki_lib_state_machine.vi"("State(s) in (\"\")"=w399) -> ("States Out"=w398:string)  [unwired: 14 in]
      }
      frame "Image: Mark droplets" {
        # "Template Separator\n(You can make a copy of, or modify, this frame)"
        n170 = Unbundle By Name(w402) -> ("Data Out Cluster.Number of droplets"=w407:i32, "Data Out Cluster.Particle Measurements"=w406:dbl[][], "Camera Cluster.Image"=w405:T1)
        n171 = for {
          N: w407 -> [_]
          tunnel: w406 -> [w419] mode=indexing
          shift-right: [w422] -> w400
          shift-left: w405 -> [w423]
          tunnel: w404 -> [w421]
          tunnel: [w420] -> w403
          w425 = u32 0 items=["Frame", "Fill"] ("Drawing Mode (Frame)")
          n172 = Index Array(array=w419) -> (element #1=w416:dbl, element #2=w415:dbl, element #3=w410:dbl)  [unwired: 4 in, 1 out]
          n173 = Divide(x=w410, y=2.0) -> (x/y=w417:dbl)
          n174 = Add(x=w416, y=w417) -> (x+y=w411:dbl)
          n175 = Subtract(x=w416, y=w417) -> (x-y=w412:dbl)
          n176 = Add(x=w415, y=w417) -> (x+y=w413:dbl)
          n177 = Subtract(x=w415, y=w417) -> (x-y=w414:dbl)
          n178 = Bundle By Name(cluster=T6 {"Left"=0, "Top"=0, "Right"=0, "Bottom"=0} ("Bounding Rectangle"), "Left"=w412, "Top"=w414, "Right"=w411, "Bottom"=w413) -> (w426:T6)
          n179 = call "IMAQ Overlay Oval"("Color"=u32 16711680, "error in (no error)"=w421, "Drawing Mode (Frame)"=w425, "Bounding Rectangle"=w426, "Image"=w423) -> ("error out"=w420:errorcluster, "Image Out"=w422:T1)  [unwired: 5 in]
        }
        n180 = Bundle By Name(cluster=w402, "Camera Cluster.Position Image Rings"=w400) -> (w401:T2)
        n181 = call <vilib>:"Add State(s) to Queue__jki_lib_state_machine.vi"("State(s) in (\"\")"=w409) -> ("States Out"=w408:string)  [unwired: 14 in]
        n182 = local write "Image"(w400) -> ()
      }
    }
    n183 = call <extravilib>:"Write.vi"("element"=w12) -> ("channel"=w8:T9)  [unwired: 1 out]
  }
  n184 = while {
    tunnel: w5 -> [w438]
    tunnel: [w437] -> w4
    shift-right: [w432] -> _
    shift-left: FALSE -> [w428]
    stop <- w435 stop-if-true
    # "Pixel analasys loop"
    n185 = call <extravilib>:"Read.vi"("channel"=w438) -> ("element"=w434:T2)  [unwired: 1 in, 1 out]
    n186 = Unbundle By Name(w434) -> ("Active"=w431:bool, "Exit"=w436:bool)
    n187 = Not(x=w428) -> (.not. x?=w429:bool)
    n188 = And(x=w429, y=w431) -> (x .and. y?=w430:bool)
    n189 = case shown="False" w430 {
      tunnel: w438 -> [_ w449]
      tunnel: i64 100 ("Sample dt (ms)") -> [_ w446]
      tunnel: [_ w445] -> w437
      tunnel: w436 -> [w440 w444]
      tunnel: [w440 w444] -> w435
      tunnel: [w439 w442] -> w432
      tunnel: w428 -> [w439 _]
      frame False {
        n190 = Wait (ms)(milliseconds to wait=u32 100) -> ()  [unwired: 1 out]
      }
      frame True {
        n191 = node-c288(w446) -> (w448:T11)  [unwired: 1 in]
        n192 = timed-loop {
          tunnel: w449 -> [w464]
          shift-right: [w465] -> _
          shift-left: errorcluster {"status"=FALSE, "code"=0, "source"=""} ("error out") -> [w466]
          timing: w448 -> [_]
          timing-out: [_] -> w447
          shift-right: [w474] -> _
          shift-left: _ -> [w475]
          tunnel: [w468] -> w445
          shift-right: [w470] -> _
          shift-left: _ -> [w471]
          tunnel: [w451] -> w442
          i -> [w456]
          stop <- w450 stop-if-true
          n193 = node-c288() -> ()  [unwired: 1 in, 1 out]
          n194 = call <extravilib>:"Read.vi"("channel"=w464) -> ("element"=w460:T2)  [unwired: 1 in, 1 out]
          n195 = Unbundle By Name(w460) -> ("Exit"=w453:bool, "Active"=w479:bool, "Data In Cluster.Number of images"=w455:i32)
          n196 = call "Data_Recollection_GCFS.vi"("error in (no error)"=w466, "cnt"=w456, "Cluster"=w460) -> ("error out"=w465:errorcluster, "Timestamp"=w462:string, "Temp"=w461:dbl, "Image Out"=w463:T1)  [unwired: 1 in]
          "Frezz Image" <- w463
          "Temperature" <- w461
          n197 = Not(x=w479) -> (.not. x?=w452:bool)
          n198 = call "Image_Pixel_Values_RE_GCFS.vi"("date/time string"=w462, "Image in"=w463, "Temperature"=w461, "Cluster"=w460) -> ("Value_Array"=w457:string[], "Freezing_points"=w458:string[], "Freezing data"=w459:bool)  [unwired: 1 out]
          n199 = Format Into String(w461) -> (resulting string=w467:string)  [unwired: 3 in, 1 out]
          n200 = xnode "Match Regular Expression"("input string"=w462, "regular expression"="_" ("search string/char (-)")) -> ("after match"=w472:string)  [unwired: 4 in, 4 out]
          n201 = Insert Into Array(array=w457, index=0, new element #1=w472, new element #2=w467) -> (w476:string[])
          n202 = Decrement(x=w455) -> (x-1=w454:i32)
          n203 = Equal?(x=w454, y=w456) -> (x = y?=w451:bool)
          n204 = Build Array (concatenate)(w458, w471) -> (w470:string[][])
          n205 = Build Array (concatenate)(w475, w476) -> (w474:string[][])
          n206 = Compound Arithmetic op=OR(w453, w452, w451) -> (w450:bool)
          n207 = Bundle By Name(cluster=T10 {"Image To Save"=refnum, "Snap timestamp"="", "Pixel values"=[], "Freezing points"=[], "FreezingData"=FALSE}, "FreezingData"=w459, "Freezing points"=w470, "Pixel values"=w474, "Snap timestamp"=w462) -> (w469:T10)
          n208 = call <extravilib>:"Write.vi"("last element? (F)"=w450, "element"=w469) -> ("channel"=w468:T14)  [unwired: 7 in, 2 out]
          n209 = node-c288() -> ()  [unwired: 1 out]
          "Data Loop" <- w456
        }
        n210 = node-c288(w447) -> ()
        n211 = property on="Done" class="Bool (strict)"("Val(Sgnl)"=w442) -> ()  [unwired: 2 in, 2 out]
      }
    }
  }
  n212 = while {
    tunnel: w5 -> [w610]
    tunnel: w4 -> [w613]
    shift-right: [w608] -> _
    shift-left: FALSE ("last element?") -> [w603]
    i -> [w611]
    stop <- w612 stop-if-true
    n213 = call <extravilib>:"Read.vi"("channel"=w610) -> ("element"=w609:T2)  [unwired: 1 in, 1 out]
    n214 = Unbundle By Name(w609) -> ("Active"=w606:bool, "Exit"=w607:bool)
    n215 = Not(x=w603) -> (.not. x?=w605:bool)
    n216 = And(x=w605, y=w606) -> (x .and. y?=w604:bool)
    n217 = case shown="False" w604 {
      tunnel: w609 -> [_ w628]
      tunnel: w613 -> [_ w623]
      tunnel: w607 -> [w616 w619]
      tunnel: [w616 w618] -> w612
      tunnel: [w614 w617] -> w608
      tunnel: w603 -> [w614 _]
      frame False {
        n218 = Wait (ms)(milliseconds to wait=u32 100) -> ()  [unwired: 1 out]
      }
      frame True {
        # "Append to file loop"
        n219 = Unbundle By Name(w628) -> ("Data In Cluster.Images.Rerun Folder path"=w627:path)
        n220 = call <extravilib>:"Read.vi"("channel"=w623) -> ("last element?"=w617:bool, "element"=w622:T10)  [unwired: 6 in, 3 out]
        n221 = Unbundle By Name(w622) -> ("FreezingData"=w621:bool, "Snap timestamp"=w624:string, "Freezing points"=w625:string[][])
        n222 = feedback #1() -> (w626:string)  [unwired: 1 in]
        n223 = feedback-in #1(w624) -> ()
        n224 = Not Equal?(x=w624, y=w626) -> (x != y?=w620:bool)
        n225 = case shown="True" w620 {
          tunnel: w627 -> [_ w632]
          tunnel: w625 -> [_ w633]
          tunnel: w621 -> [_ w634]
          tunnel: w619 -> [w629 w631]
          tunnel: [w629 w631] -> w618
          frame False {
            n226 = Wait (ms)(milliseconds to wait=u32 100) -> ()  [unwired: 1 out]
          }
          frame True {
            n227 = case shown="False" w634 {
              tunnel: w633 -> [_ w636]
              tunnel: w632 -> [_ w635]
              frame False {
              }
              frame True {
                n228 = call "Save_Files_GCFS.vi"("Enum"=enum16{"Freezing_Data", "Sample_Data"}."Freezing_Data", "Array"=w636, "file path (use dialog)"=w635) -> ()  [unwired: 2 in, 2 out]
              }
            }
          }
        }
      }
    }
    "Save loop" <- w611
  }
